vi "getErrorCode.vi"(8 "error in (no error)":errorcluster, 9 "code":u16, 10 "errorType":T1, 11 "CoolerSerialCommand in":refnum<class "CoolerSerialCommand.lvclass">) -> (0 "error out":errorcluster, 2 "errorCode":u16, 3 "CoolerSerialCommand out":refnum<class "CoolerSerialCommand.lvclass">)   [LabVIEW 2016, in "CoolerSerialCommand.lvclass"]
uses:
  CoolerSerialCommand.lvclass
  typedefs/errorType.ctl
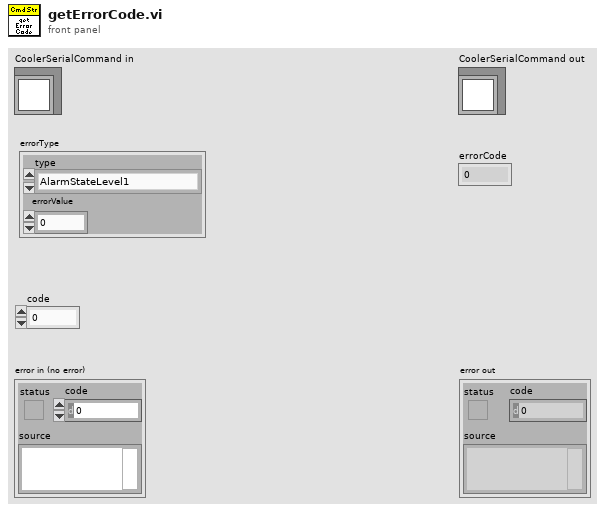
[diagram p1: front panel]
types:
  T1 = typedef "errorType.ctl" = cluster{"type":enum16{"AlarmStateLevel1", "AlarmStateLevel21", "AlarmStateLevel22", "WarningStateLevel1"}, "errorValue":u16}
  T2 = enum16{"AlarmStateLevel1", "AlarmStateLevel21", "AlarmStateLevel22", "WarningStateLevel1"}
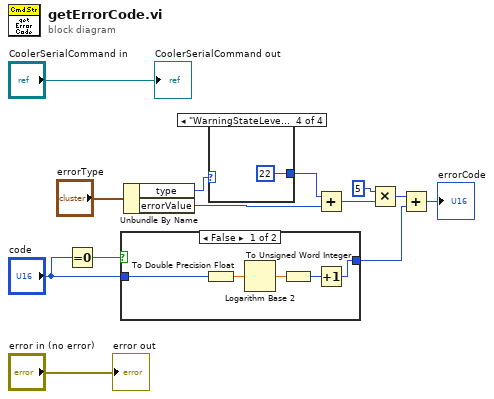
[diagram p0: block diagram]
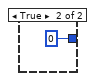
[diagram p2: hidden frame]
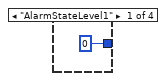
[diagram p3: hidden frame]
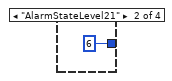
[diagram p4: hidden frame]
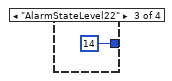
[diagram p5: hidden frame]
diagram:
  n1 = Equal To 0?(x="code") -> (x = 0?=w7:bool)
  n2 = case shown="False" w7 {
    tunnel: [w18 u16 0] -> w2
    tunnel: "code" -> [w14 _]
    frame False {
      n3 = To Double Precision Float(number=w14) -> (double precision float=w15:dbl)
      n4 = Logarithm Base 2(1:w15) -> (0:w16:dbl)
      n5 = To Unsigned Word Integer(number=w16) -> (unsigned 16bit integer=w17:u16)
      n6 = Increment(x=w17) -> (x+1=w18:u16)
    }
    frame True {
    }
  }
  n7 = Unbundle By Name("errorType") -> ("type"=w11:T2, "errorValue"=w10:u16)
  n8 = case shown="\"WarningStateLevel1\"" w11 {
    tunnel: [u16 0 u16 6 u16 14 u16 22] -> w9
    frame "AlarmStateLevel1" {
    }
    frame "AlarmStateLevel21" {
    }
    frame "AlarmStateLevel22" {
    }
    frame "WarningStateLevel1" {
    }
  }
  n9 = Add(x=w9, y=w10) -> (x+y=w5:u16)
  n10 = Multiply(x=u16 5, y=w5) -> (x*y=w3:u16)
  n11 = Add(x=w3, y=w2) -> (x+y=→"errorCode":u16)
  "error out" <- "error in (no error)"
  "CoolerSerialCommand out" <- "CoolerSerialCommand in"
